vi "MW_Display_Python_Detect_Device.vi"(0 "session in":refnum<k35>, 5 "module path":path, 11 "error in":errorcluster) -> (4 "session out":refnum<k35>, 6 "module path out":path, 13 "Device Information":string[](array[string]), 14 "Number of Device Detected":i32, 15 "error out":errorcluster)   [LabVIEW 2023]
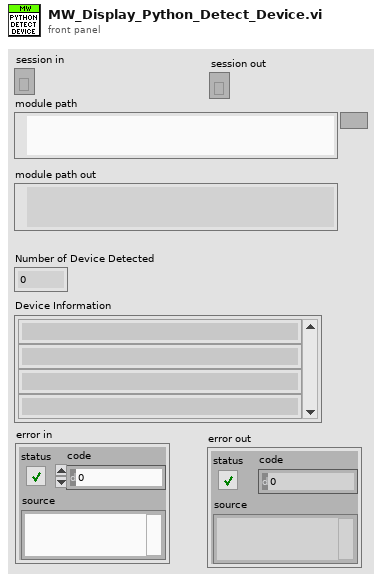
[diagram p1: front panel]
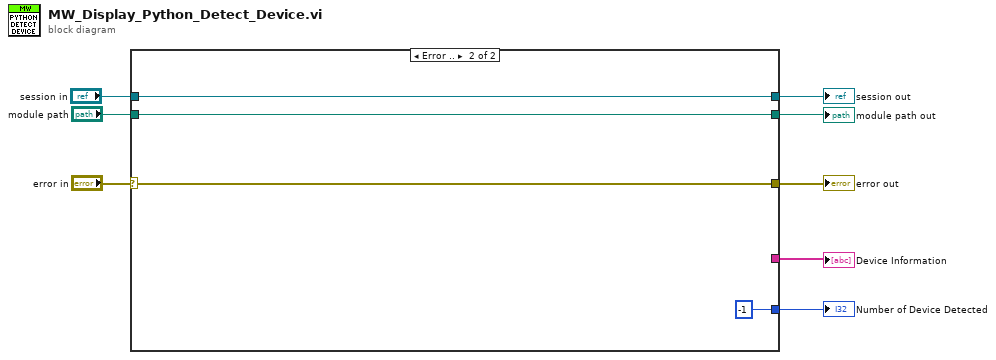
[diagram p0: block diagram]
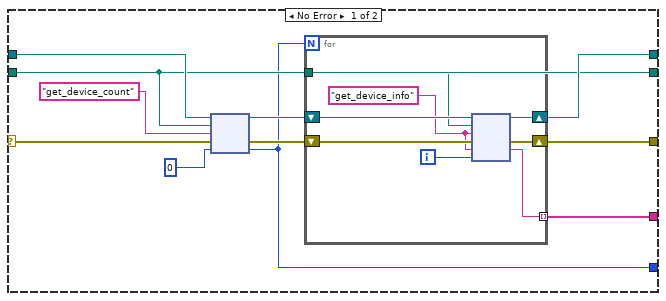
[diagram p2: hidden frame]
diagram:
  n1 = case shown="Error .." "error in" {
    selector: "error in" -> [w16 w31]
    tunnel: [w10 -1] -> w8
    tunnel: "session in" -> [w17 w29]
    tunnel: "module path" -> [w11 w28]
    tunnel: [w12 w31] -> w6
    tunnel: [w13 w29] -> w5
    tunnel: [w11 w28] -> w3
    tunnel: [w9 _] -> w1
    frame No Error {
      n2 = node(w17, w11, "get_device_count" ("function name"), w16, 0) -> (w14:refnum<k35>, w15:errorcluster, w10:i32)  [unwired: 2 out]
      n3 = for {
        N: w10 -> [_]
        tunnel: w11 -> [w23]
        shift-right: [w24] -> w12
        shift-left: w15 -> [w27]
        shift-right: [w25] -> w13
        shift-left: w14 -> [w26]
        tunnel: [w20] -> w9 mode=indexing
        i -> [w22]
        w21 = "get_device_info" ("function name")
        n4 = node(w26, w23, w21, w27, w21, w22) -> (w25:refnum<k35>, w24:errorcluster, w20:string)  [unwired: 1 in, 2 out]
      }
    }
    frame Error {
    }
  }
  "Number of Device Detected" <- w8
  "error out" <- w6
  "session out" <- w5
  "module path out" <- w3
  "Device Information" <- w1
